vi "Test.vi"   [LabVIEW 2014]
types:
  T1 = typedef "SessionPrimary.ctl" = cluster{"setup":u8, "subject_id":i32, "session_start_time":dbl}
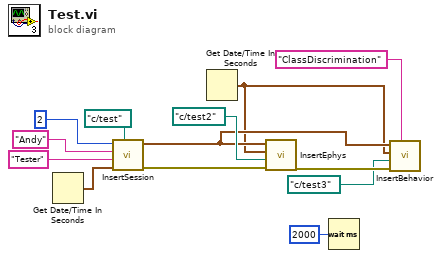
[diagram p0: block diagram]
diagram:
  n1 = Get Date/Time In Seconds() -> (seconds since 1Jan1904=w12:timestamp)
  n2 = call "InsertSession.vi"("session_path"=path "c:/test", "error in (no error)"=w12, "experimenter"="Tester", "subject"="Andy", "setup"=u8 2) -> ("error out"=w13:errorcluster, "SessionPK"=w6:T1)  [unwired: 5 in]
  n3 = Get Date/Time In Seconds() -> (seconds since 1Jan1904=w4:timestamp)
  n4 = call "InsertEphys.vi"("error in (no error)"=w13, "ephys_path"=path "c:/test2", "ephys_start_time"=w4, "connection reference"=w6) -> ("error out"=w5:errorcluster)  [unwired: 6 in, 1 out]
  n5 = Wait (ms)(milliseconds to wait=u32 2000) -> ()  [unwired: 1 out]
  n6 = call "InsertBehavior.vi"("exp_type"="ClassDiscrimination", "error in (no error)"=w5, "beh_path"=path "c:/test3", "beh_start_time"=w4, "connection reference"=w6) -> ()  [unwired: 5 in, 2 out]
